vi "Calculate Latency Statistics.vi"(10 "Stimulus Onsets (s)":dbl[](array[numeric]), 11 "Response Onsets (s)":dbl[](array[numeric])) -> (1 "Latency sd":dbl, 2 "Latency mean":dbl, 3 "Latency (s)":dbl[](array[numeric]))   [LabVIEW 2016]
uses:
  <vilib>/Analysis/NI_AALBase.lvlib
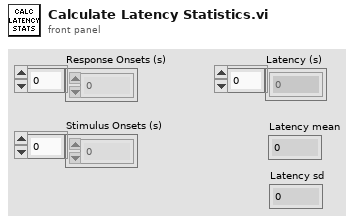
[diagram p1: front panel]
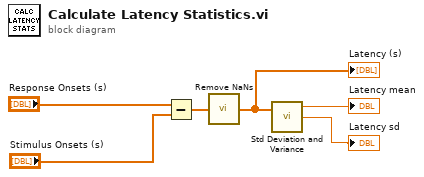
[diagram p0: block diagram]
diagram:
  n1 = Subtract(x="Response Onsets (s)", y="Stimulus Onsets (s)") -> (x-y=w4:dbl[])
  n2 = call <userlib>:"Remove NaNs.vi"("Data in"=w4) -> ("Data Out"=w1:dbl[])  [unwired: 5 in, 1 out]
  "Latency (s)" <- w1
  n3 = call <vilib>:"Std Deviation and Variance.vi"("X"=w1) -> ("mean"=→"Latency mean":dbl, "standard deviation"=→"Latency sd":dbl)  [unwired: 1 in, 1 out]
